vi "Idle_Timer_RW.vi"(7 "R/W":enum16{"Write", "Read"}(ring)=enum."Read", 8 "error in":errorcluster, 11 "Idle Timer In":T1={"OP10"=0.2, "OP20"=0.2, "OP30"=0.2, "OP40"=0.2, "OP50"=0.2, "OP60"=0.2} {"OP60" min=0.1 max=9999999.0; "OP50" min=0.1 max=9999999.0; "OP40" min=0.1 max=9999999.0; "OP30" min=0.1 max=9999999.0; "OP20" min=0.1 max=9999999.0; "OP10" min=0.1 max=9999999.0}) -> (0 "error out":errorcluster, 3 "Idle Timer Out":T1={"OP10"=0.2, "OP20"=0.2, "OP30"=0.2, "OP40"=0.2, "OP50"=0.2, "OP60"=0.2} {"OP60" min=0.1 max=9999999.0; "OP50" min=0.1 max=9999999.0; "OP40" min=0.1 max=9999999.0; "OP30" min=0.1 max=9999999.0; "OP20" min=0.1 max=9999999.0; "OP10" min=0.1 max=9999999.0})   [LabVIEW 2020]
uses:
  Controls/Idle_Timer.ctl
  Controls/Idle_Timer_disp.ctl
  MS SQL/MS_Global.vi
panel:
  out "Path Out":path
  # "Idle Timer"
  # "Idle Timer"
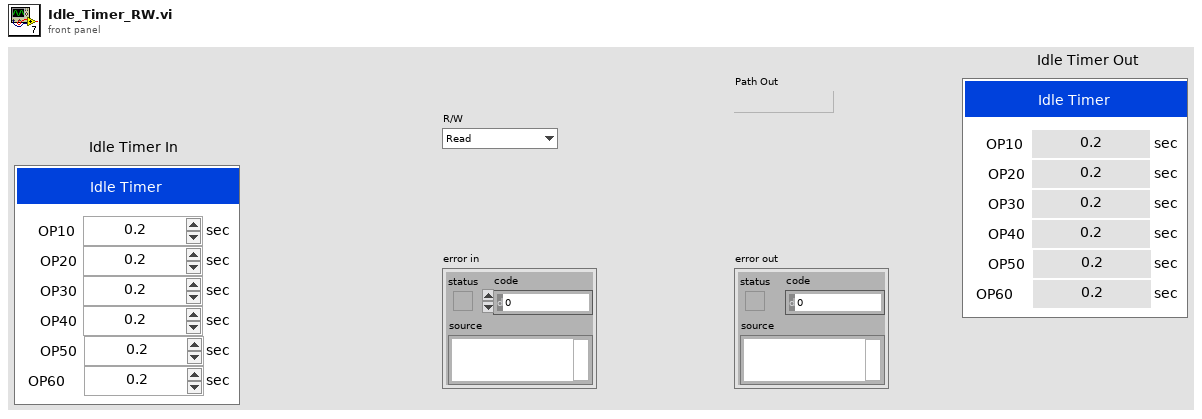
[diagram p1: front panel]
types:
  T1 = typedef "Idle_Timer.ctl" = cluster{"OP10":T2, "OP20":T2, "OP30":T2, "OP40":T2, "OP50":T2, "OP60":T2}
  T2 = typedef "Idle_Timer_disp.ctl" = dbl
  T3 = enum16{"open", "replace", "create", "open or create", "replace or create", "replace or create with confirmation"}
  T4 = cluster{"Data Path":path, "Calibration Path":path, "Settings Path":path, "Script Path":path, "DAQ Support":path, "Reporting Desktop":path, "Help":path}
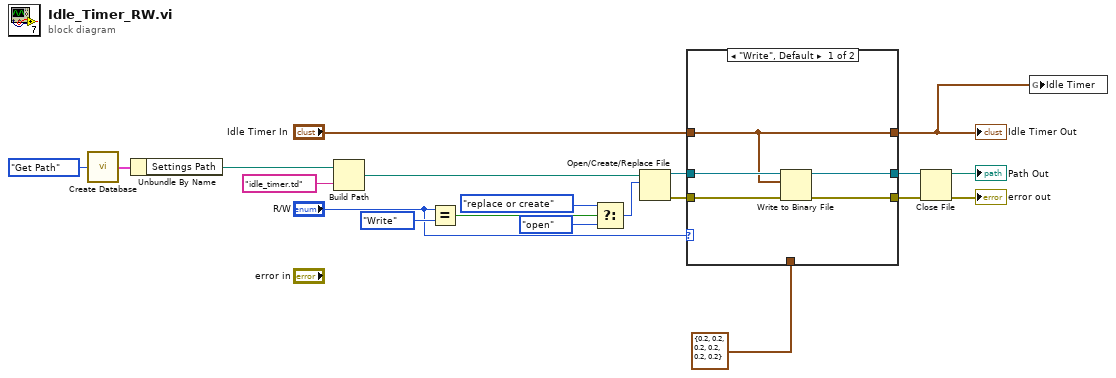
[diagram p0: block diagram]
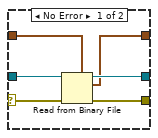
[diagram p3: hidden frame]
diagram:
  n1 = call <userlib>:"Create Database.vi"("Get/Create"=enum16{"Get Path", "Create Path"}."Get Path") -> ("Path Out"=w16:T4)  [unwired: 13 in, 1 out]
  n2 = Unbundle By Name(w16) -> ("Settings Path"=w20:path)
  n3 = Build Path(base path=w20, name or relative path="idle_timer.td" ("File Name")) -> (appended path=w18:path)
  n4 = Equal?(x="R/W", y=enum16{"Write", "Read"}."Write" ("R/W 2")) -> (x = y?=w13:bool)
  n5 = Select(t=T3."replace or create", s=w13, f=T3."open" ("operation (0:open)")) -> (s? t:f=w10:T3)
  n6 = Open/Create/Replace File(file path (use dialog)=w18, operation (0:open)=w10) -> (refnum out=w9:refnum<file>, error out=w7:errorcluster)  [unwired: 4 in, 1 out]
  n7 = case shown="\"Write\", Default" "R/W" {
    tunnel: w9 -> [w25 w32]
    tunnel: w7 -> [w24 w27]
    tunnel: "Idle Timer In" -> [w21 w29]
    tunnel: [w23 w31] -> w4
    tunnel: [w22 w30] -> w5
    tunnel: [w21 w28] -> w2
    tunnel: T1 {"OP10"=0.2, "OP20"=0.2, "OP30"=0.2, "OP40"=0.2, "OP50"=0.2, "OP60"=0.2} ("Idle Timer In") -> [_ w26]
    frame "Write", Default {
      n8 = Write to Binary File(file (use dialog)=w25, data=w21, error in=w24) -> (refnum out=w23:refnum<file>, error out=w22:errorcluster)  [unwired: 3 in, 1 out]
    }
    frame "Read" {
      n9 = case shown="Error" w27 {
        selector: w27 -> [w33 w40]
        tunnel: w32 -> [w38 w41]
        tunnel: [w37 w41] -> w31
        tunnel: [w36 w40] -> w30
        tunnel: w29 -> [w35 _]
        tunnel: [w34 w39] -> w28
        tunnel: w26 -> [_ w39]
        frame No Error {
          n10 = Read from Binary File(5:w35, 8:w33, 11:w38) -> (0:w36:errorcluster, 2:w34:T1, 3:w37:refnum<file>)  [unwired: 3 in, 1 out]
        }
        frame Error {
        }
      }
    }
  }
  "Idle Timer Out" <- w2
  n11 = Close File(refnum=w4, error in=w5) -> (path=→"Path Out":path, error out=→"error out":errorcluster)
  n12 = global write "MS_Global.vi" "Idle Timer"(w2) -> ()
